vi "VI Tree.vi"   [LabVIEW 2020, in "Template - Spectrum Analyzer.lvlib"]
doc: "This is the instrument driver for the <INSTRUMENT NAME>. The VI Tree displays all the user-callable VIs of the instrument driver in an organized table."
uses:
  <instrlib>/_Template - Spectrum Analyzer/Template - Spectrum Analyzer.lvlib
  <instrlib>/_Template - Spectrum Analyzer/Public/Configure/Configure Frequency (Start Stop).vi
panel:
  # "(c) 2014 <Enter Company Name Here>.  ALL RIGHTS RESERVED."
  # "SEE DIAGRAM\nFOR VI TREE."
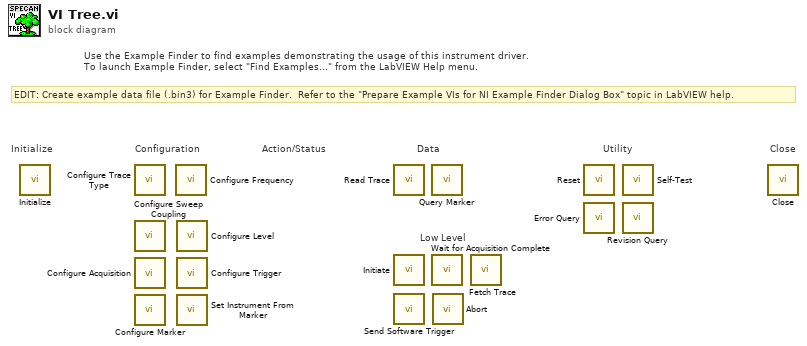
[diagram p0: block diagram]
diagram:
  # "EDIT: Create example data file (.bin3) for Example Finder.  Refer to the \"Prepare Example VIs for NI Example Finder Dialog Box\" topic in LabVIEW help."
  # "Low Level"
  # "Use the Example Finder to find examples demonstrating the usage of this instrument driver.\nTo launch Example Finder, select \"Find Examples...\" from the LabVIEW Help menu."
  # "Configuration"
  # "Utility"
  # "Data"
  # "Action/Status"
  # "Close"
  # "Initialize"
  n1 = call <instrlib>:"Initialize.vi"() -> ()  [unwired: 10 in, 2 out]
  n2 = call <instrlib>:"Configure Trace Type.vi"() -> ()  [unwired: 10 in, 2 out]
  n3 = call <instrlib>:"Configure Sweep Coupling.vi"() -> ()  [unwired: 10 in, 2 out]
  n4 = call <instrlib>:"Configure Acquisition.vi"() -> ()  [unwired: 10 in, 2 out]
  n5 = call <instrlib>:"Configure Marker.vi"() -> ()  [unwired: 10 in, 2 out]
  n6 = call-poly <instrlib>:"Configure Frequency.vi"() -> ()  [unwired: 10 in, 2 out]
  n7 = call <instrlib>:"Configure Level.vi"() -> ()  [unwired: 10 in, 2 out]
  n8 = call <instrlib>:"Configure Trigger.vi"() -> ()  [unwired: 10 in, 2 out]
  n9 = call <instrlib>:"Set Instrument From Marker.vi"() -> ()  [unwired: 10 in, 2 out]
  n10 = call <instrlib>:"Read Trace.vi"() -> ()  [unwired: 9 in, 3 out]
  n11 = call <instrlib>:"Initiate.vi"() -> ()  [unwired: 10 in, 2 out]
  n12 = call <instrlib>:"Send Software Trigger.vi"() -> ()  [unwired: 10 in, 2 out]
  n13 = call <instrlib>:"Query Marker.vi"() -> ()  [unwired: 8 in, 4 out]
  n14 = call <instrlib>:"Wait for Acquisition Complete.vi"() -> ()  [unwired: 10 in, 2 out]
  n15 = call <instrlib>:"Abort.vi"() -> ()  [unwired: 10 in, 2 out]
  n16 = call <instrlib>:"Fetch Trace.vi"() -> ()  [unwired: 7 in, 5 out]
  n17 = call <instrlib>:"Reset.vi"() -> ()  [unwired: 10 in, 2 out]
  n18 = call <instrlib>:"Error Query.vi"() -> ()  [unwired: 8 in, 4 out]
  n19 = call <instrlib>:"Self-Test.vi"() -> ()  [unwired: 8 in, 4 out]
  n20 = call <instrlib>:"Revision Query.vi"() -> ()  [unwired: 8 in, 4 out]
  n21 = call <instrlib>:"Close.vi"() -> ()  [unwired: 11 in, 1 out]
